vi "Status Updated.vi"(8 "error in (no error)":errorcluster, 10 "Status":string, 11 "Module ID":i32=-1) -> (0 "error out":errorcluster)   [LabVIEW 2014, in "ConfigurableQMH.lvlib"]
doc: "Send the Status Updated event to any VI registered to listen to events from the owning module.\n_____\nBased on Delacor QMH Project Template 4.0.0.47."
uses:
  ConfigurableQMH.lvlib
  Status Updated Argument--cluster.ctl
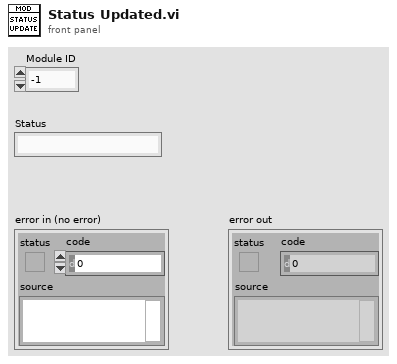
[diagram p1: front panel]
types:
  T1 = typedef "ConfigurableQMH.lvlib/Status Updated Argument--cluster.ctl" = cluster{"Status":string, "Module ID":i32}
  T2 = typedef "ConfigurableQMH.lvlib/Broadcast Events--cluster.ctl" = cluster{"Module Did Init":refnum<user-event>, "Status Updated":refnum<user-event>, "Error Reported":refnum<user-event>, "Module Did Stop":refnum<user-event>, "Update Module Execution Status":refnum<user-event>, "Module Configuration":refnum<user-event>}
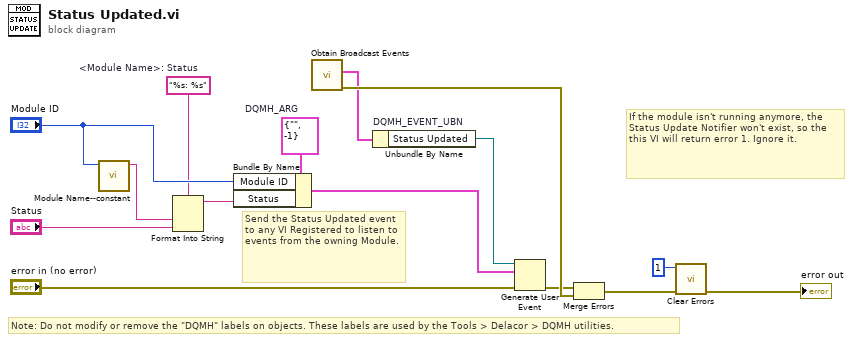
[diagram p0: block diagram]
diagram:
  w7 = "%s: %s"  # <Module Name>: Status
  w10 = T1 {"Status"="", "Module ID"=-1}  # DQMH_ARG
  # "If the module isn't running anymore, the Status Update Notifier won't exist, so the this VI will return error 1. Ignore it."
  # "Note: Do not modify or remove the \"DQMH\" labels on objects. These labels are used by the Tools > Delacor > DQMH utilities."
  # "Send the Status Updated event to any VI Registered to listen to events from the owning Module."
  n1 = call "Module Name--constant.vi"("Module ID"="Module ID") -> ("Module Name"=w6:string)  [unwired: 10 in]
  n2 = Format Into String(format string=w7, w6, "Status") -> (resulting string=w4:string)  [unwired: 2 in, 1 out]
  n3 = Bundle By Name(cluster=w10, "Module ID"="Module ID", "Status"=w4) -> (w9:T1)
  n4 = call "Obtain Broadcast Events.vi"() -> ("error out"=w14:errorcluster, "ConfigurableQMH Broadcast Events"=w12:T2)  [unwired: 10 in]
  n5 = Unbundle By Name "DQMH_EVENT_UBN"(w12) -> ("Status Updated"=w11:refnum<user-event>)
  n6 = Generate User Event(user event=w11, event data cluster=w9, error in="error in (no error)") -> (error out=w13:errorcluster)  [unwired: 1 in, 1 out]
  n7 = Merge Errors(w13, w14) -> (w2:errorcluster)
  n8 = call <vilib>:"Clear Errors.vi"("error in (no error)"=w2, "specific error code to clear (0: all)"=1) -> ("error out"=→"error out":errorcluster)  [unwired: 4 in, 1 out]
